vi "Do.vi"(8 "error in (no error)":errorcluster, 10 "Actor In":refnum<class "Actor.lvclass">, 11 "Message in":refnum<class "Message.lvclass">) -> (0 "error out":errorcluster, 1 "Stop Actor":bool, 2 "Actor Out":refnum<class "Actor.lvclass">)   [LabVIEW 2020, in "Artifex.lvlib" / "Message.lvclass"]
uses:
  Message.lvclass
  Actor/Actor.lvclass
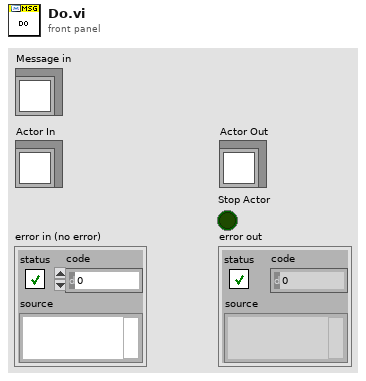
[diagram p1: front panel]
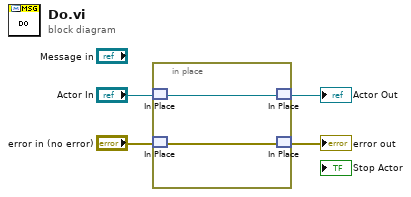
[diagram p0: block diagram]
diagram:
  n1 = in-place {
    n2 = in-place-match #1("Actor In") -> (w5:refnum<class "Actor.lvclass">)
    n3 = in-place-match #2("error in (no error)") -> (w6:errorcluster)
    n4 = in-place-match #1(w5) -> (→"Actor Out":refnum<class "Actor.lvclass">)
    n5 = in-place-match #2(w6) -> (→"error out":errorcluster)
  }
